vi "2182A and 2400 Combined Measuring.vi"() -> ()   [LabVIEW 2022 SP3]
uses:
  <vilib>/Analysis/baseanly.llb/Mean (DBL).vi
  Keithley 24XX Sweep and Acquire Measurements Folder/Public/Data/Read (Single Point).vi
  <instrlib>/Keithley 2182/Keithley 2182.lvlib
  Keithley 24XX Sweep and Acquire Measurements Folder/Keithley 24XX.lvlib
  <vilib>/Analysis/NI_AALBase.lvlib
panel:
  out "2182A error out":errorcluster
  out "2400 error out":errorcluster
  in  "Resistance Measurement":T1(tab)
  out "New file path 2":path
  in  "Folder to save file to":path=path "C:/Users/PNA User/Documents/NZ LabView Project/LabViewData"
  in  "2400":T2={"Baud Rate"=9600, "Parity"=0, "Data Bits"=8, "Stop Bits"=10, "Flow Control"=0, "VISA resource name"="SourceMeter"} {"Flow Control" items=["None", "XON/XOFF", "RTS/CTS", "XON/XOFF & RTS/CTS", "DTR/DSR", "XON/XOFF & DTR/DSR"]; "Stop Bits" items=["1.0"=10, "1.5"=15, "2.0"=20]; "Data Bits" items=["7"=7, "8"=8]; "Parity" items=["None", "Odd", "Even", "Mark", "Space"]; "Baud Rate" items=["300"=300, "600"=600, "1200"=1200, "2400"=2400, "4800"=4800, "9600"=9600, "19200"=19200]}
  in  "Current (µA)":dbl=350.0
  in  "Source Mode  (0: Voltage)":u16(ring)=1 items=["Voltage", "Current"]
  in  "Compliance  Level (0.1)":dbl=42.0
  in  "2182A":T2={"Baud Rate"=9600, "Parity"=0, "Data Bits"=8, "Stop Bits"=10, "Flow Control"=0, "VISA resource name"="NanoVoltMeter"} {"Flow Control" items=["None", "XON/XOFF", "RTS/CTS", "XON/XOFF & RTS/CTS", "DTR/DSR", "XON/XOFF & DTR/DSR"]; "Stop Bits" items=["1.0"=10, "1.5"=15, "2.0"=20]; "Data Bits" items=["7"=7, "8"=8]; "Parity" items=["None", "Odd", "Even", "Mark", "Space"]; "Baud Rate" items=["300"=300, "600"=600, "1200"=1200, "2400"=2400, "4800"=4800, "9600"=9600, "19200"=19200]}
  in  "Measurement (0: Voltage Channel 1) 2":i32(ring) items=["Voltage Channel 1", "Voltage Channel 2", "Temperature Channel 1", "Temperature Channel 2"]
  in  "Number of experiments to run":i32=1
  in  "Delay After Taking Reading (ms)":dbl
  in  "Enable Current Auto Range (T:Enable)":bool=TRUE
  in  "Current Manual Range (1.0)":dbl=1.0
  in  "Integration Rate (5)":dbl=5.0
  in  "Range Value (12)":dbl=12.0
  in  "Voltage Resolution (8)":i32=8
  in  "Delay Before Taking Reading (ms)":dbl=5.0
  out "Current Supplied By 2400":sgl[](array[numeric])
  out "Voltage Read By 2182":dbl[](array[numeric])
  out "Resistance Calculated":dbl[](array[numeric])
  out "Mean of Resistance Over All Experiments":dbl
  out "Mean of Voltage Over All Experiments":dbl
  out "Mean of Current Over All Experiments":dbl
  out "Standard Deviation Voltage":dbl
  out "Standard Deviation Resistance":dbl
  out "Standard Deviation Current":dbl
  # "If all values entered correctly but doesn't work consider restarting PC"
  # "2400"
  # "2182"
  # "Basic"
  # "42V recomended"
  # "2400"
  # "2182"
  # "Ext"
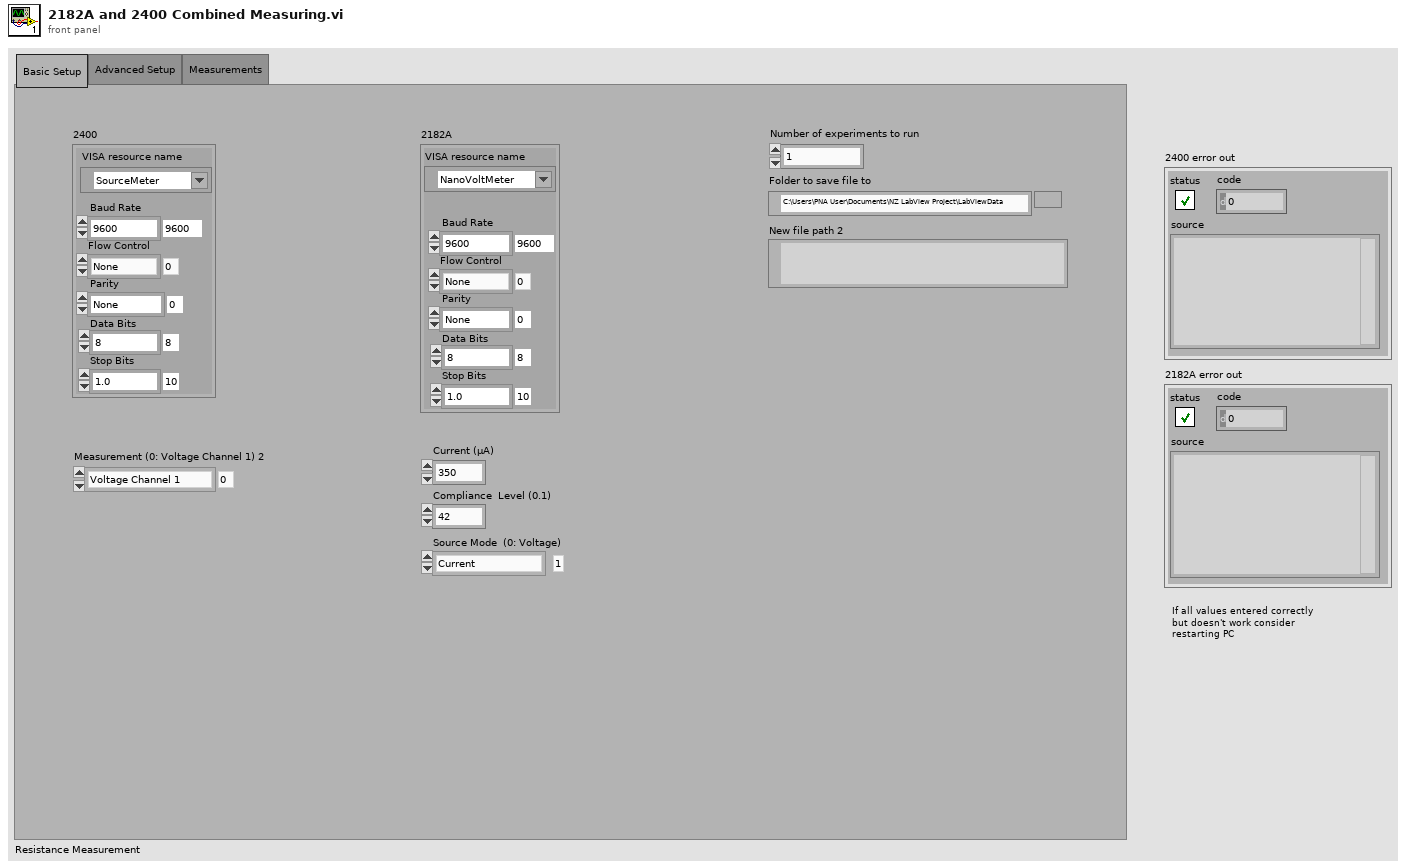
[diagram p1: front panel]
types:
  T1 = enum32{"Basic Setup", "Advanced Setup", "Measurements"}
  T2 = cluster{"Baud Rate":u32, "Parity":u16, "Data Bits":u16, "Stop Bits":u16, "Flow Control":u16, "VISA resource name":refnum<visa-resource-name>}
  T3 = enum16{"open", "replace", "create", "open or create", "replace or create", "replace or create with confirmation"}
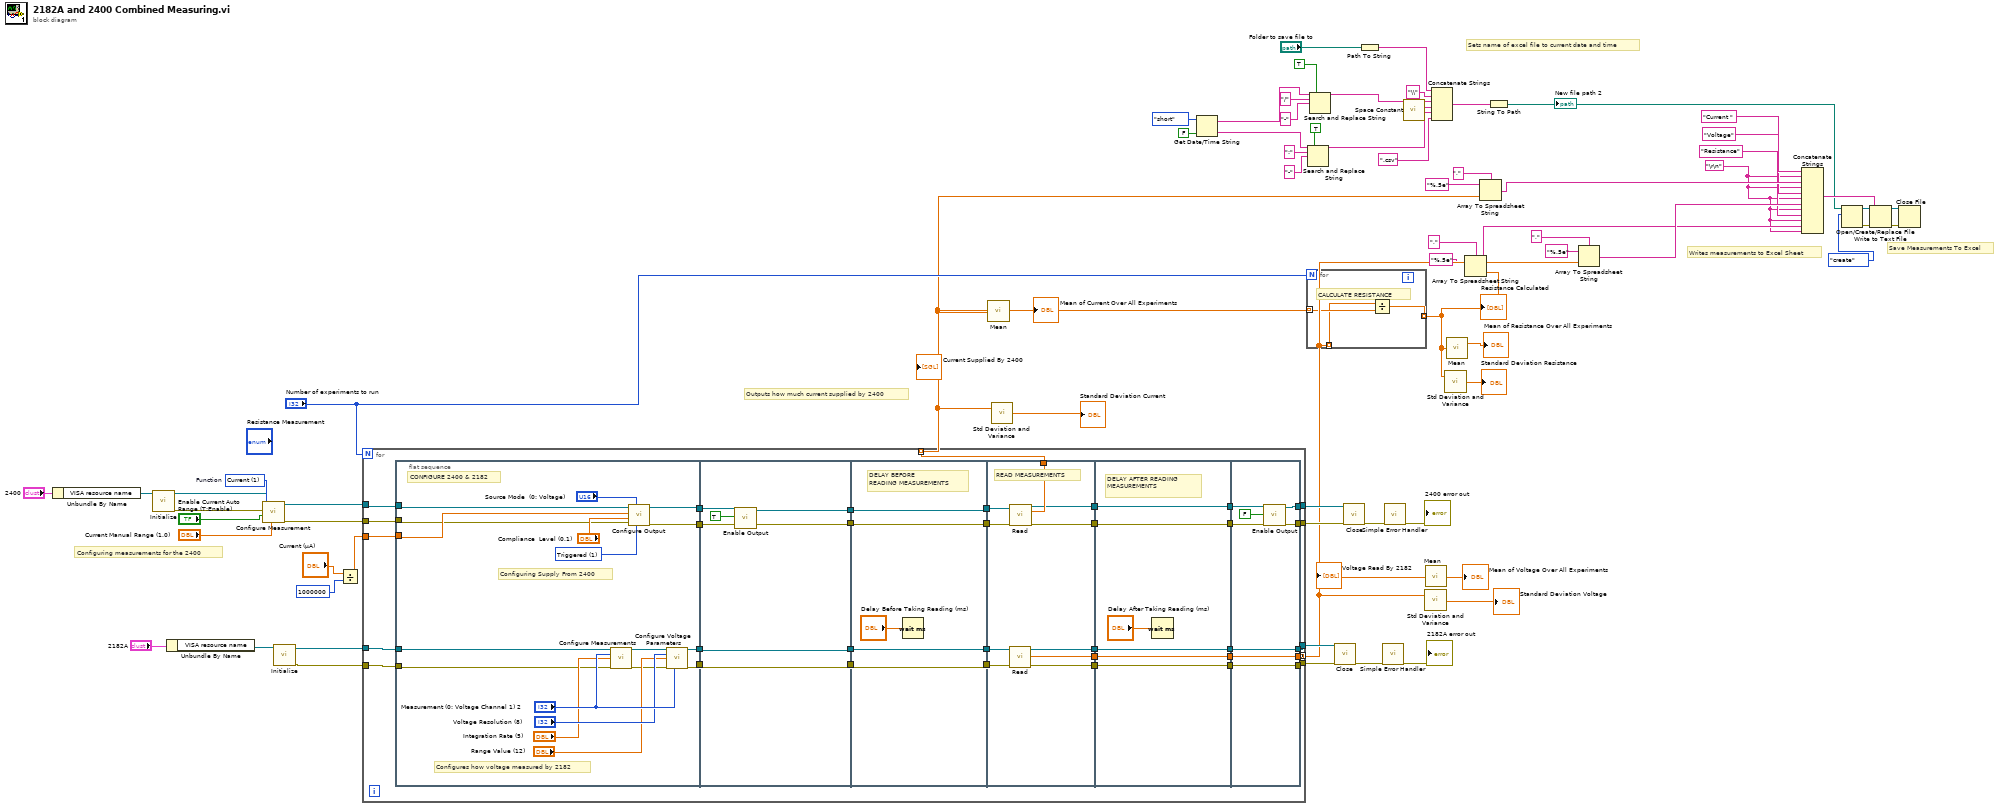
[diagram p0: block diagram]
diagram:
  w1 = "\r\n"
  w72 = u16 1 items=["Volts", "Current", "Resistance"]  # Function
  # "Writes measurements to Excel Sheet"
  # "Sets name of excel file to current date and time"
  # "Save Measurements To Excel"
  # "Outputs how much current supplied by 2400"
  # "Configuring measurements for the 2400"
  n1 = Unbundle By Name("2400") -> ("VISA resource name"=w68:refnum<visa-resource-name>)
  n2 = call <instrlib>:"Initialize.vi"("VISA resource name"=w68) -> ("error out"=w61:errorcluster, "VISA resource name out"=w62:refnum<visa-resource-name>)  [unwired: 9 in]
  n3 = Unbundle By Name("2182A") -> ("VISA resource name"=w59:refnum<visa-resource-name>)
  n4 = call "Configure Measurement.vi"("Manual Range (1.0)"="Current Manual Range (1.0)", "error in (no error)"=w61, "Enable Auto Range (T:Enable)"="Enable Current Auto Range (T:Enable)", "Function (0: Volts)"=w72, "VISA resource name"=w62) -> ("error out"=w65:errorcluster, "VISA resource name out"=w66:refnum<visa-resource-name>)  [unwired: 5 in]
  n5 = call <instrlib>:"Initialize.vi"("VISA resource name"=w59) -> ("error out"=w63:errorcluster, "VISA resource name out"=w64:refnum<visa-resource-name>)  [unwired: 9 in]
  n6 = Divide(x="Current (µA)", y=1000000) -> (x/y=w56:dbl)
  n7 = for {
    N: "Number of experiments to run" -> [_]
    tunnel: w66 -> [w103]
    tunnel: w65 -> [w104]
    tunnel: w64 -> [w102]
    tunnel: w63 -> [w101]
    tunnel: w56 -> [w105]
    tunnel: [w100] -> w14 mode=indexing
    tunnel: [w99] -> w11 mode=concatenating
    tunnel: [w98] -> w54
    tunnel: [w97] -> w53
    tunnel: [w74] -> w52
    tunnel: [w73] -> w51
    n8 = flat-sequence {
      tunnel: w105 -> [w114]
      tunnel: w104 -> [w113]
      tunnel: w103 -> [w112]
      tunnel: w102 -> [w111]
      tunnel: w101 -> [w110]
      tunnel: [w109] -> w89
      tunnel: [w108] -> w87
      tunnel: [w107] -> w80
      tunnel: [w106] -> w79
      tunnel: w89 -> [w130]
      tunnel: [w130] -> w88
      tunnel: w87 -> [w129]
      tunnel: [w129] -> w86
      tunnel: w80 -> [w127]
      tunnel: w79 -> [w126]
      tunnel: [w125] -> w77
      tunnel: [w124] -> w75
      tunnel: w88 -> [w135]
      tunnel: [w135] -> w96
      tunnel: w86 -> [w134]
      tunnel: [w134] -> w95
      tunnel: [w133] -> w78
      tunnel: w77 -> [w133]
      tunnel: [w132] -> w76
      tunnel: w75 -> [w132]
      tunnel: w96 -> [w145]
      tunnel: w95 -> [w144]
      tunnel: [w143] -> w100
      tunnel: [w142] -> w94
      tunnel: [w141] -> w93
      tunnel: [w140] -> w92
      tunnel: [w139] -> w91
      tunnel: [w138] -> w90
      tunnel: w78 -> [w137]
      tunnel: w76 -> [w136]
      tunnel: w94 -> [w151]
      tunnel: w93 -> [w150]
      tunnel: w92 -> [w149]
      tunnel: w91 -> [w148]
      tunnel: w90 -> [w147]
      tunnel: [w151] -> w85
      tunnel: [w150] -> w84
      tunnel: [w149] -> w83
      tunnel: [w148] -> w82
      tunnel: [w147] -> w81
      tunnel: [w157] -> w97
      tunnel: [w158] -> w98
      tunnel: [w159] -> w99
      tunnel: w85 -> [w159]
      tunnel: w84 -> [w158]
      tunnel: w83 -> [w157]
      tunnel: w82 -> [w155]
      tunnel: w81 -> [w154]
      tunnel: [w153] -> w74
      tunnel: [w152] -> w73
      frame #0 {
        w121 = u16 1 items=["Immediate", "Triggered"] ("Output Type  (0: Immediate)")
        # "CONFIGURE 2400 & 2182"
        # "Configures how voltage measured by 2182"
        # "Configuring Supply From 2400"
        n9 = call <instrlib>:"Configure Measurements.vi"("VISA resource name"=w111, "Measurement (0: Voltage Channel 1)"="Measurement (0: Voltage Channel 1) 2", "Integration Rate (5)"="Integration Rate (5)", "error in (no error)"=w110) -> ("VISA resource name out"=w115:refnum<visa-resource-name>, "error out"=w116:errorcluster)  [unwired: 10 in]
        n10 = call "Configure Output.vi"("Output Type  (0: Immediate)"=w121, "Source Mode  (0: Voltage)"="Source Mode  (0: Voltage)", "error in (no error)"=w113, "Compliance  Level (0.1)"="Compliance  Level (0.1)", "Output Level (0)"=w114, "VISA resource name"=w112) -> ("error out"=w106:errorcluster, "VISA resource name out"=w107:refnum<visa-resource-name>)  [unwired: 4 in]
        n11 = call <instrlib>:"Configure Voltage Parameters.vi"("VISA resource name"=w115, "Measurement (1: Voltage Channel 1)"="Measurement (0: Voltage Channel 1) 2", "Voltage Resolution (8)"="Voltage Resolution (8)", "Range Value (12)"="Range Value (12)", "error in (no error)"=w116) -> ("VISA resource name out"=w108:refnum<visa-resource-name>, "error out"=w109:errorcluster)  [unwired: 9 in]
      }
      frame #1 {
        n12 = call "Enable Output.vi"("error in (no error)"=w126, "Enable Output (T: Enable)"=TRUE, "VISA resource name"=w127) -> ("error out"=w124:errorcluster, "VISA resource name out"=w125:refnum<visa-resource-name>)  [unwired: 7 in]
      }
      frame #2 {
        # "DELAY BEFORE \nREADING MEASUREMENTS"
        n13 = Wait (ms)(milliseconds to wait="Delay Before Taking Reading (ms)") -> ()  [unwired: 1 out]
      }
      frame #3 {
        # "READ MEASUREMENTS"
        n14 = call <instrlib>:"Read.vi"("error in (no error)"=w145, "VISA resource name"=w144) -> ("error out"=w140:errorcluster, "Measurements"=w142:dbl[], "VISA resource name out"=w141:refnum<visa-resource-name>)  [unwired: 6 in, 1 out]
        n15 = call-poly <instrlib>:"Read.vi"("VISA resource name"=w137, "error in (no error)"=w136) -> ("VISA resource name out"=w139:refnum<visa-resource-name>, "Current"=w143:sgl, "error out"=w138:errorcluster)  [unwired: 7 in, 4 out]
      }
      frame #4 {
        # "DELAY AFTER READING MEASUREMENTS"
        n16 = Wait (ms)(milliseconds to wait="Delay After Taking Reading (ms)") -> ()  [unwired: 1 out]
      }
      frame #5 {
        n17 = call "Enable Output.vi"("error in (no error)"=w154, "Enable Output (T: Enable)"=FALSE, "VISA resource name"=w155) -> ("error out"=w152:errorcluster, "VISA resource name out"=w153:refnum<visa-resource-name>)  [unwired: 7 in]
      }
    }
  }
  "Current Supplied By 2400" <- w14
  "Voltage Read By 2182" <- w11
  n18 = call-poly <vilib>:"Mean.vi"("X"=w14) -> ("mean"=→"Mean of Current Over All Experiments":dbl)  [unwired: 1 out]
  n19 = call <vilib>:"Std Deviation and Variance.vi"("X"=w14) -> ("standard deviation"=→"Standard Deviation Current":dbl)  [unwired: 1 in, 2 out]
  n20 = Get Date/Time String(date format (0)=enum16{"short", "long", "abbreviated"}."short", want seconds? (F)=FALSE) -> (date string=w30:string, time string=w35:string)  [unwired: 1 in]
  n21 = for {
    N: "Number of experiments to run" -> [_]
    tunnel: w14 -> [w162] mode=indexing
    tunnel: [w161] -> w8 mode=indexing
    tunnel: w11 -> [w160] mode=indexing
    # "CALCULATE RESISTANCE"
    n22 = Divide(x=w160, y=w162) -> (x/y=w161:dbl)
  }
  "Resistance Calculated" <- w8
  n23 = Search and Replace String(replace all?=TRUE ("replace all? (F)"), input string=w35, search string=":" ("replace string (\"\")"), replace string="-" ("replace string (\"\")")) -> (result string=w39:string)  [unwired: 4 in, 3 out]
  n24 = Search and Replace String(replace all?=TRUE, input string=w30, search string="/" ("replace string (\"\")"), replace string="-" ("replace string (\"\")")) -> (result string=w29:string)  [unwired: 4 in, 3 out]
  n25 = call <instrlib>:"Close.vi"("error in (no error)"=w53, "VISA resource name"=w54) -> ("error out"=w55:errorcluster)  [unwired: 9 in]
  n26 = call <instrlib>:"Close.vi"("error in (no error)"=w51, "VISA resource name"=w52) -> ("error out"=w67:errorcluster)  [unwired: 9 in]
  n27 = Path To String(path="Folder to save file to") -> (string=w43:string)
  n28 = call <vilib>:"Simple Error Handler.vi"("error in (no error)"=w55) -> ("error out"=→"2182A error out":errorcluster)  [unwired: 4 in, 4 out]
  n29 = call <vilib>:"Simple Error Handler.vi"("error in (no error)"=w67) -> ("error out"=→"2400 error out":errorcluster)  [unwired: 4 in, 4 out]
  n30 = call <vilib>:"Space Constant.vi"() -> ("String"=w38:string)
  n31 = call <vilib>:"Std Deviation and Variance.vi"("X"=w11) -> ("standard deviation"=→"Standard Deviation Voltage":dbl)  [unwired: 1 in, 2 out]
  n32 = call-poly <vilib>:"Mean.vi"("X"=w11) -> ("mean"=→"Mean of Voltage Over All Experiments":dbl)  [unwired: 1 out]
  n33 = Concatenate Strings "Concatenate Strings"(w43, "\\" ("string"), w29, w38, w39, ".csv" ("string")) -> (w41:string)
  n34 = call <vilib>:"Std Deviation and Variance.vi"("X"=w8) -> ("standard deviation"=→"Standard Deviation Resistance":dbl)  [unwired: 1 in, 2 out]
  n35 = call-poly <vilib>:"Mean.vi"("X"=w8) -> ("mean"=→"Mean of Resistance Over All Experiments":dbl)  [unwired: 1 out]
  n36 = Array To Spreadsheet String(delimiter (Tab)=",", array=w8, 3:"%.5e") -> (spreadsheet string=w2:string)
  n37 = Array To Spreadsheet String(delimiter (Tab)=",", array=w14, 3:"%.5e") -> (spreadsheet string=w6:string)
  n38 = String To Path(string=w41) -> (path=w15:path)
  "New file path 2" <- w15
  n39 = Array To Spreadsheet String(delimiter (Tab)=",", array=w11, 3:"%.5e") -> (spreadsheet string=w4:string)
  n40 = Concatenate Strings("Current ", w1, w6, w1, "Voltage", w1, w4, w1, "Resistance", w1, w2, w1) -> (w22:string)
  n41 = Open/Create/Replace File(file path (use dialog)=w15, operation (0:open)=T3."create") -> (refnum out=w25:refnum<file>, error out=w26:errorcluster)  [unwired: 4 in, 1 out]
  n42 = Write to Text File(file (use dialog)=w25, text=w22, error in=w26) -> (refnum out=w23:refnum<file>, error out=w24:errorcluster)  [unwired: 1 in, 1 out]
  n43 = Close File(refnum=w23, error in=w24) -> ()  [unwired: 2 out]
